vi "Cleanup.vi"(8 "error in (no error)":errorcluster, 11 "Stop High Pressure Wash in":refnum<class "Stop High Pressure Wash.lvclass">) -> (0 "error out":errorcluster, 3 "Stop High Pressure Wash out":refnum<class "Stop High Pressure Wash.lvclass">)   [LabVIEW 2019, in "Stop High Pressure Wash.lvclass"]
uses:
  <vilib>/gpm_packages/@cs/Car-wash/Source/Process Steps/Stop High Pressure Wash/Stop High Pressure Wash.lvclass
  <vilib>/gpm_packages/@cs/Car-wash/Source/iProcess Step Model/iProcess Step Model/iProcess Step Model.lvclass
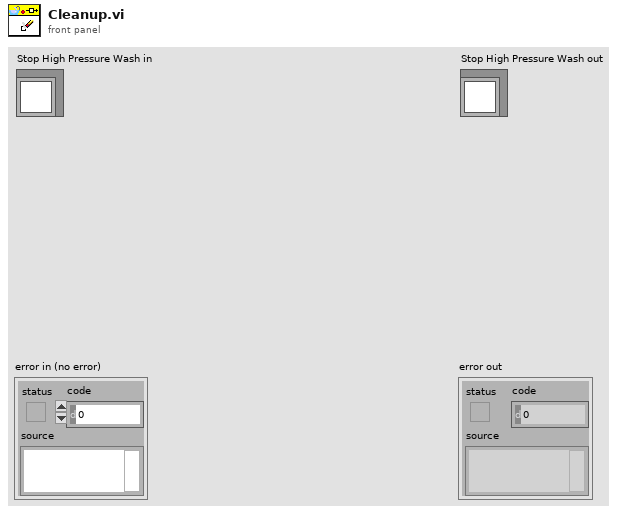
[diagram p1: front panel]
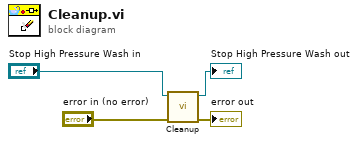
[diagram p0: block diagram]
diagram:
  n1 = call-parent "Cleanup.vi"("error in (no error)"="error in (no error)", "iProcess Step Model in"="Stop High Pressure Wash in") -> ("error out"=→"error out":errorcluster, "iProcess Step Model out"=→"Stop High Pressure Wash out":refnum<class "Stop High Pressure Wash.lvclass">)  [unwired: 8 in]
